vi "capture.vi"(8 "error in (no error)":errorcluster, 9 "Session In":T2="cam3", 10 "Image Name":string="img", 11 "Timeout (ms)":i32=5000) -> (0 "error out 4":errorcluster, 3 "Image":T1(plugin-control))   [LabVIEW 2017]
uses:
  <vilib>/userdefined/High Color/IMAQdx.ctl
  <vilib>/vision/driver/IMAQdx.llb/IMAQdx Camera Control Mode.ctl
  <vilib>/vision/driver/IMAQdx.llb/IMAQdx Acquisition Mode.ctl
  <vilib>/vision/driver/NI_Vision_Acquisition_Software.lvlib
panel:
  out "error out 3":errorcluster
  out "error out 2":errorcluster
  out "error out":errorcluster
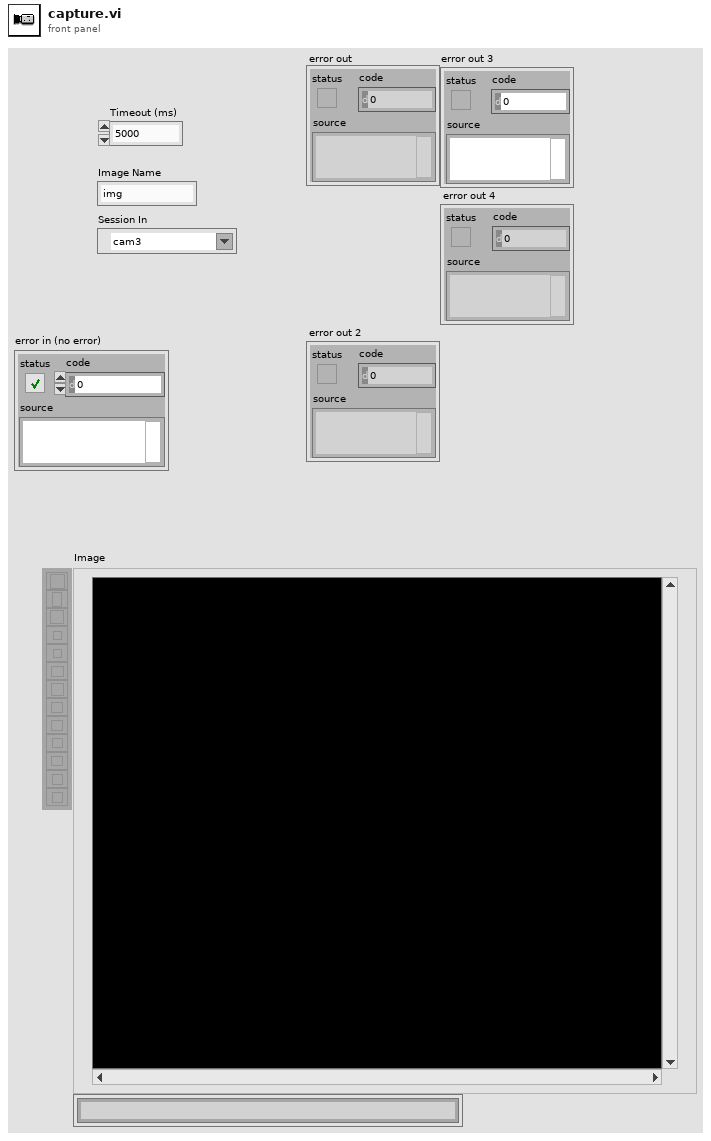
[diagram p1: front panel]
types:
  T1 = typedef "IMAQ Image.ctl" = refnum<image>
  T2 = typedef "IMAQdx.ctl" = refnum<k21>
  T3 = typedef "NI_Vision_Acquisition_Software.lvlib/IMAQdx Acquisition Mode.ctl" = enum32{"One Shot", "Continuous"}
  T4 = typedef "NI_Vision_Acquisition_Software.lvlib/IMAQdx Camera Control Mode.ctl" = enum32{"Controller", "Listener"}
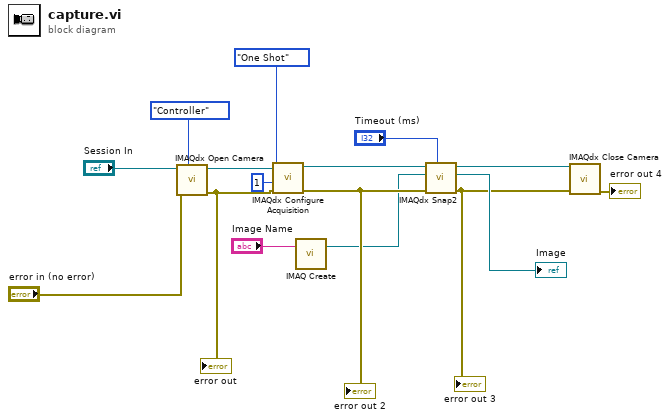
[diagram p0: block diagram]
diagram:
  n1 = call <vilib>:"IMAQdx Open Camera.vi"("Camera Control Mode"=IMAQdx_Camera_Control_Mode."Controller", "error in"="error in (no error)", "Session In"="Session In") -> ("error out"=w12:errorcluster, "Session Out"=w13:T2)  [unwired: 7 in]
  "error out" <- w12
  n2 = call <vilib>:"IMAQdx Configure Acquisition.vi"("error in"=w12, "Number of Buffers"=u32 1, "Continuous?"=IMAQdx_Acquisition_Mode."One Shot", "Session In"=w13) -> ("error out"=w8:errorcluster, "Session Out"=w9:T2)  [unwired: 6 in]
  "error out 2" <- w8
  n3 = call "IMAQ Create"("Image Name"="Image Name") -> ("New Image"=w7:T1)  [unwired: 4 in, 1 out]
  n4 = call <vilib>:"IMAQdx Snap2.vi"("Timeout (ms)"="Timeout (ms)", "error in"=w8, "Image In"=w7, "Session In"=w9) -> ("error out"=w4:errorcluster, "Image Out"=→"Image":T1, "Session Out"=w5:T2)  [unwired: 5 in]
  "error out 3" <- w4
  n5 = call <vilib>:"IMAQdx Close Camera.vi"("error in"=w4, "Session In"=w5) -> ("error out"=→"error out 4":errorcluster)  [unwired: 9 in]
